vi "Read parameters.vi"(8 "error in (no error)":errorcluster, 11 "Telegram Class in":refnum<class "Telegram Class.lvclass">) -> (0 "error out":errorcluster, 2 "parameters":T1={"database_directory"="", "use_file_database"=TRUE, "use_chat_info_database"=TRUE, "use_message_database"=TRUE, "use_secret_chats"=TRUE, "api_id"=0, "api_hash"="", "system_language_code"="en", "device_model"="Desktop", "application_version"="0.1", "enable_storage_optimizer"=TRUE}, 3 "Telegram Class out":refnum<class "Telegram Class.lvclass">)   [LabVIEW 2015, in "Telegram Library.lvlib" / "Telegram Class.lvclass"]
doc: "Created IvanLis by LabVIEW Portal\nProfile: http://labviewportal.org/memberlist.php?mode=viewprofile&u=987\neMail: IvanLisanov@gMail.com\nTelegram: https://t.me/IvanLis"
uses:
  Telegram Class.lvclass
  TypeDef/TDLib Parameters.ctl
  Telegram Class.lvclass/Telegram Class.ctl
  Telegram Library.lvlib
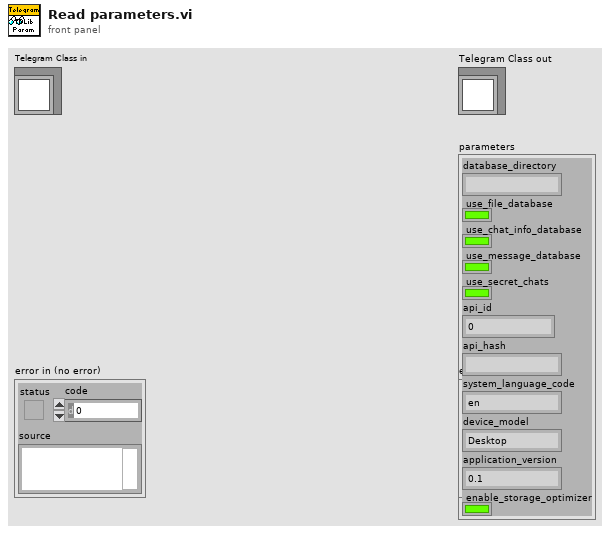
[diagram p1: front panel]
types:
  T1 = typedef "Telegram Library.lvlib/TDLib Parameters.ctl" = cluster{"database_directory":string, "use_file_database":bool, "use_chat_info_database":bool, "use_message_database":bool, "use_secret_chats":bool, "api_id":i32, "api_hash":string, "system_language_code":string, "device_model":string, "application_version":string, "enable_storage_optimizer":bool}
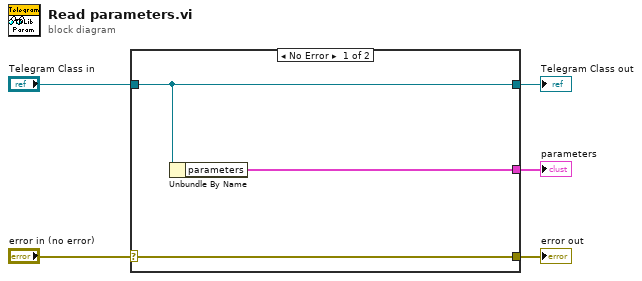
[diagram p0: block diagram]
diagram:
  n1 = case shown="No Error" "error in (no error)" {
    selector: "error in (no error)" -> [w8 w9]
    tunnel: [w8 w9] -> w4
    tunnel: [w7 w10] -> w2
    tunnel: "Telegram Class in" -> [w7 w10]
    tunnel: [w6 _] -> w1
    frame No Error {
      n2 = Unbundle By Name(w7) -> ("parameters"=w6:T1)
    }
    frame Error {
    }
  }
  "error out" <- w4
  "Telegram Class out" <- w2
  "parameters" <- w1
